vi "spot_gen_ver2.vi"(0 "amp":u32, 5 "input valid":bool, 7 "data index":u16, 9 "peak":bool, 11 "reciver_params":T1) -> (4 "PDW":u64, 6 "output valid":bool, 15 "erprr out":bool)   [LabVIEW 2021]
uses:
  FPGA/reciver params.ctl
  <vilib>/rvi/Memory/Memory_Emulation/nirvimemoryFastEmulation.vi
  <vilib>/rvi/Memory/Memory_Emulation/nirvimemoryEmulation.vi
  <vilib>/rvi/Emulation/niFpgaEmulationIsFPGAContextNoSignature.vi
  <vilib>/rvi/DataTransferAndStorage/Container/Common/niFpgaContainerGetUniqueNameForEmu.vi
  <vilib>/rvi/Emulation/niFpgaProcessEmulError.vi
  <vilib>/rvi/Emulation/niFpgaSctlEmulationGetInTimedLoop.vi
  <vilib>/rvi/errors/nirviReportUnexpectedCaseInternalError (U32).vi
  <vilib>/rvi/FXPMathLib/basic elements/FxpAddSub/XNode/nifxpmath_AddSub.xnode
  <vilib>/rvi/DataTransferAndStorage/Container/XNode/niFpgaContainer.xnode
  <vilib>/rvi/FXPMathLib/sim/FxpSim.dll
  <vilib>/rvi/FXPMathLib/FxpAdd/XNode/nifxpmath_Add.xnode
  <vilib>/rvi/FXPMathLib/FxpSub/XNode/nifxpmath_Sub.xnode
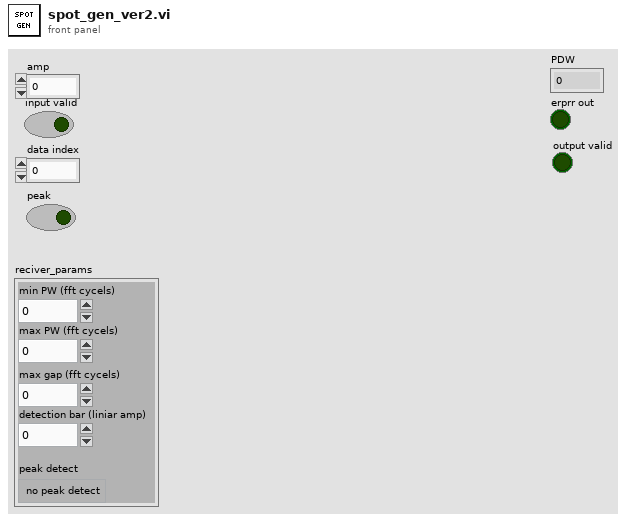
[diagram p1: front panel]
types:
  T1 = typedef "reciver params.ctl" = cluster{"min PW (fft cycels)":u16, "max PW (fft cycels)":u16, "max gap (fft cycels)":u8, "detection bar (liniar amp)":fxp<+,64,63>, "peak detect":bool}
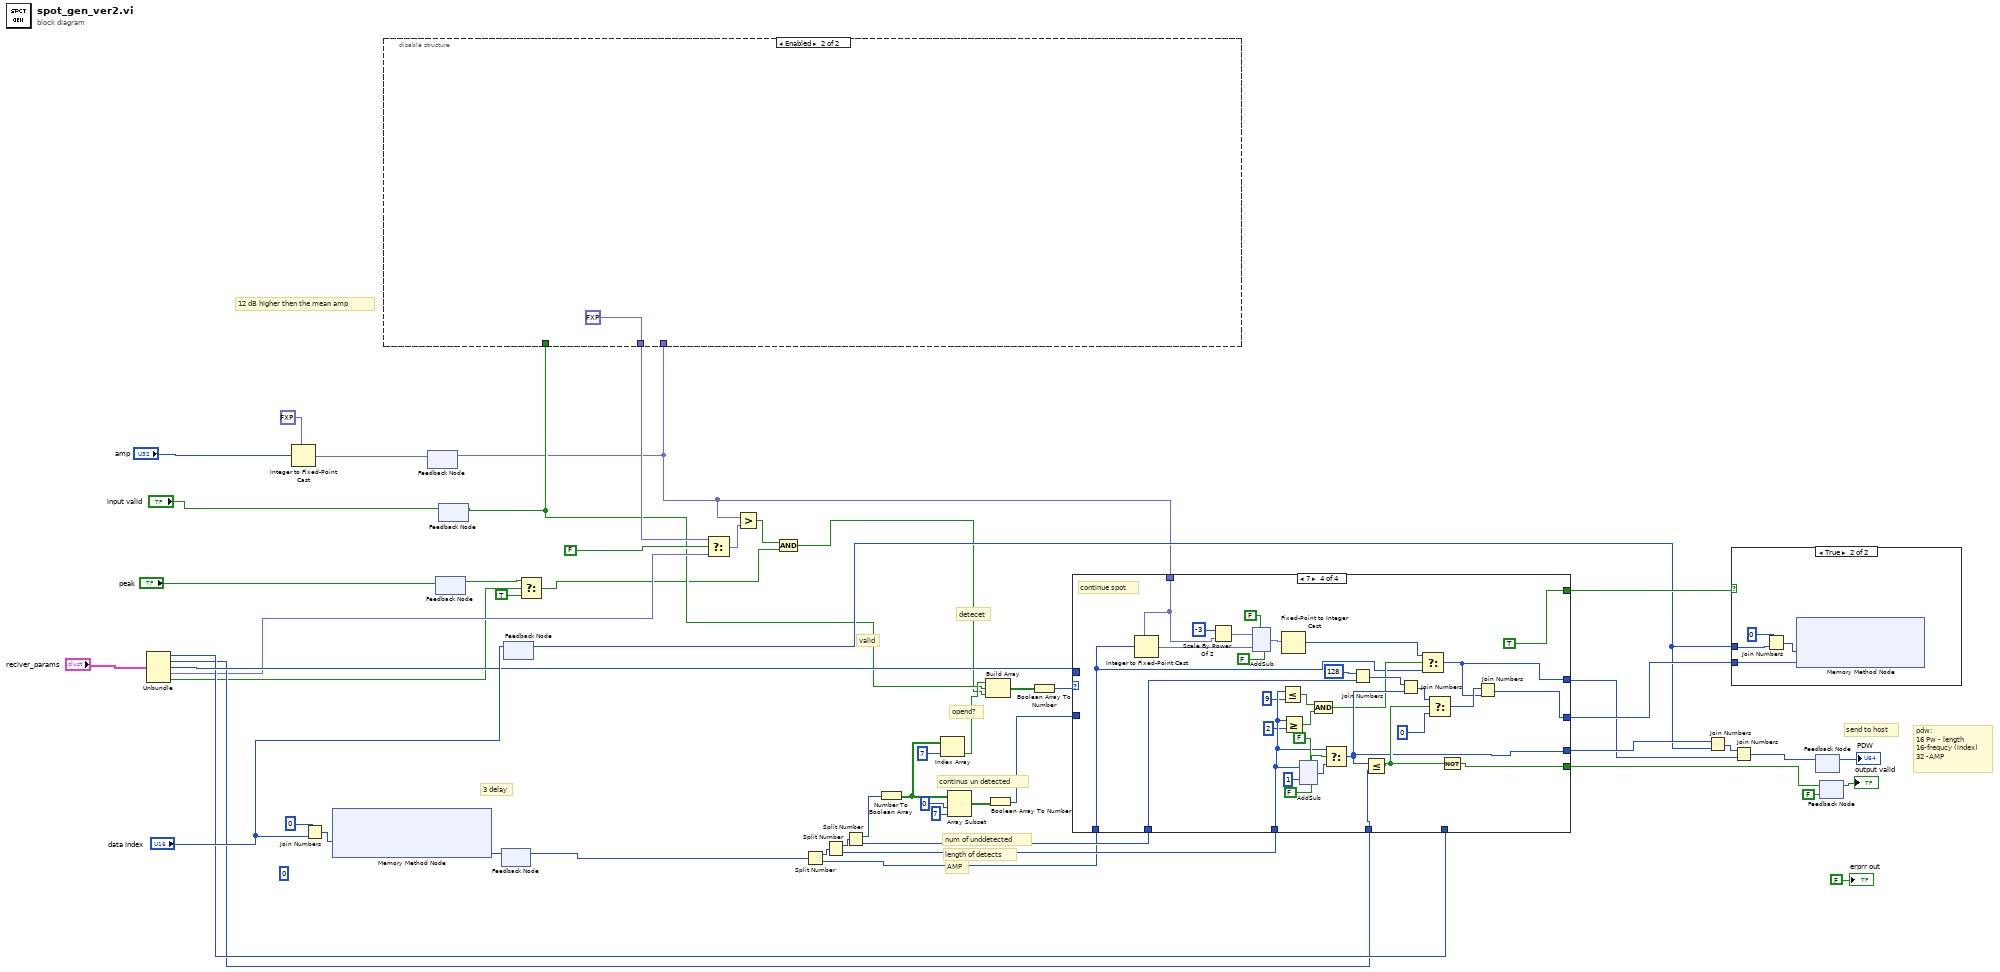
[diagram p0: block diagram]
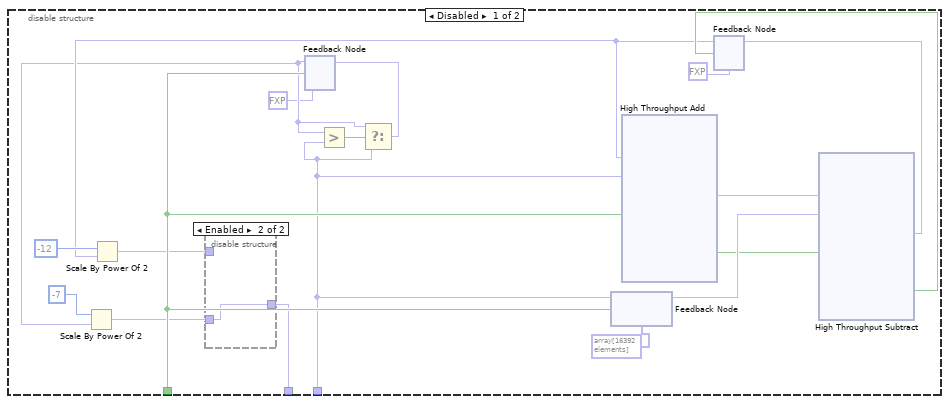
[diagram p2: hidden frame]
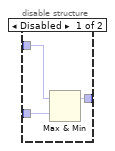
[diagram p3: hidden frame]
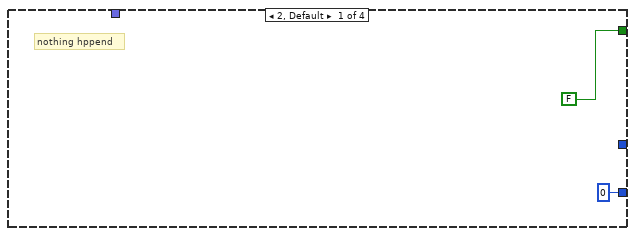
[diagram p5: hidden frame]
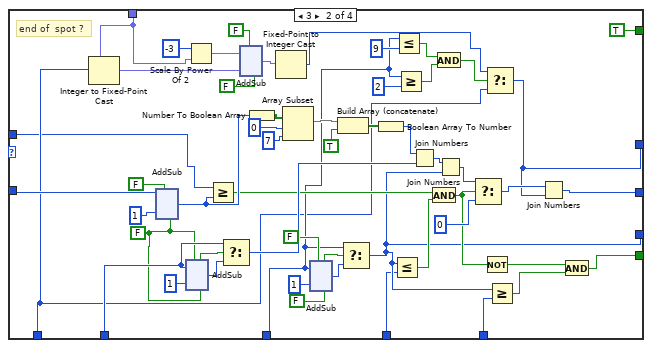
[diagram p6: hidden frame]
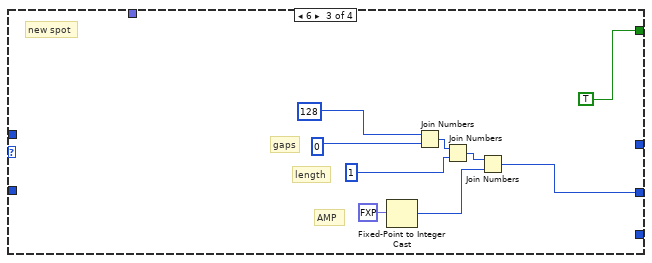
[diagram p7: hidden frame]
diagram:
  (unwired) u16 0 ("data index 2")
  # "12 dB higher then the mean amp"
  # "3 delay"
  # "AMP"
  # "pdw:\n16 Pw - length\n16-frequcy (index)\n32 -AMP"
  # "send to host"
  # "continus un detected"
  # "num of unddetected"
  # "length of detects"
  # "opend?"
  # "valid"
  # "detecet"
  n1 = Unbundle("reciver_params") -> ("min PW (fft cycels)"=w19:u16, "max PW (fft cycels)"=w18:u16, "max gap (fft cycels)"=w20:u8, "detection bar (liniar amp)"=w17:fxp<+,64,63>, "peak detect"=w1:bool)
  n2 = Integer to Fixed-Point Cast(fixed-point type=fxp<+,32,31> 0.0 ("magnitude"), integer="amp") -> (fixed-point=w6:fxp<+,32,31>)
  n3 = Join Numbers(hi=u16 0, lo="data index") -> ((hi.lo)=w24:u32)
  n4 = xnode ("Memory Method Node")("Address"=w24) -> ("Data"=w28:u64)  [unwired: 1 in, 1 out]
  n5 = feedback #1() -> (w10:fxp<+,32,31>)  [unwired: 1 in]
  n6 = feedback-in #1(w6) -> ()
  n7 = feedback #2() -> (w3:bool)  [unwired: 1 in]
  n8 = feedback-in #2("peak") -> ()
  n9 = feedback #3() -> (w11:bool)  [unwired: 1 in]
  n10 = disable-structure shown="Enabled" {
    disable-tunnel: w11 -> [w64 _]
    disable-tunnel: [w58 fxp<+,32,31> 0.0 ("magnitude")] -> w14
    disable-tunnel: w10 -> [w54 _]
    frame Disabled {
      n11 = feedback #4(fxp<+,32,31> 0.0 ("magnitude")) -> (w59:fxp<+,32,31>)
      n12 = Scale By Power Of 2(n=i8 -7 ("x"), x=w59) -> (x*2^n=w57:fxp<+,32,31>)
      n13 = Greater?(x=w59, y=w54) -> (0:w63:bool)
      n14 = Select(t=w59, s=w63, f=w54) -> (s? t:f=w61:fxp<+,32,31>)
      n15 = feedback-in #4(w61, w64) -> ()
      n16 = feedback #5(fxp<+,32,31>[] array[16392 elements]) -> (w70:fxp<+,32,31>)
      n17 = feedback-in #5(w54, w64) -> ()
      n18 = feedback #6(fxp<+,32,31> 0.0 ("s")) -> (w62:fxp<+,47,46>)
      n19 = Scale By Power Of 2(n=i8 -12 ("x"), x=w62) -> (x*2^n=w56:fxp<+,47,46>)
      n20 = disable-structure shown="Enabled" {
        disable-tunnel: [w75 w76] -> w58
        disable-tunnel: w57 -> [w74 w76]
        disable-tunnel: w56 -> [w73 _]
        frame Disabled {
          n21 = Max & Min(x=w73, y=w74) -> (max(x,y)=w75:fxp<+,47,46>)  [unwired: 1 out]
        }
        frame Enabled {
        }
      }
      n22 = xnode "High Throughput Add"("x"=w62, "y"=w54, "input valid"=w64) -> ("x+y"=w69:fxp<+,47,46>, "output valid"=w65:bool)  [unwired: 1 in, 1 out]
      n23 = xnode "High Throughput Subtract"("x"=w69, "y"=w70, "input valid"=w65) -> ("x-y"=w68:fxp<+,47,46>, "output valid"=w66:bool)  [unwired: 1 in, 1 out]
      n24 = feedback-in #6(w68, w66) -> ()
    }
    frame Enabled {
    }
  }
  n25 = feedback-in #3("input valid") -> ()
  n26 = feedback #7() -> (w27:u64)  [unwired: 1 in]
  n27 = feedback-in #7(w28) -> ()
  n28 = feedback #8() -> (w30:u16)  [unwired: 1 in]
  n29 = feedback-in #8("data index") -> ()
  n30 = Select(t=w3, s=w1, f=TRUE) -> (s? t:f=w4:bool)
  n31 = Select(t=w14, s=FALSE, f=w17) -> (s? t:f=w15:fxp<+,64,63>)
  n32 = Greater?(x=w10, y=w15) -> (0:w9:bool)
  n33 = And(x=w9, y=w4) -> (x .and. y?=w8:bool)
  n34 = Split Number(x=w27) -> (hi(x)=w34:u32, lo(x)=w33:u32)
  n35 = Split Number(x=w34) -> (hi(x)=w53:u16, lo(x)=w44:u16)
  n36 = Split Number(x=w53) -> (hi(x)=w52:u8, lo(x)=w41:u8)
  n37 = Number To Boolean Array(number=w52) -> (Boolean array=w46:bool[])
  n38 = Index Array(array=w46, index=7) -> (element=w35:bool)
  n39 = Array Subset(array=w46, index=0, length=7) -> (w49:bool[])
  n40 = Build Array(w35, w11, w8) -> (w48:bool[])
  n41 = Boolean Array To Number(Boolean array=w49) -> (number=w43:u8)
  n42 = Boolean Array To Number(Boolean array=w48) -> (number=w47:u8)
  n43 = case shown="7" w47 {
    tunnel: w44 -> [_ w87 _ w363]
    tunnel: w43 -> [_ w129 _ _]
    tunnel: [u64 0 ("Data") w99 w349 w367] -> w42
    tunnel: [FALSE TRUE TRUE TRUE] -> w40
    tunnel: w41 -> [_ w119 _ w382]
    tunnel: [_ w102 _ w376] -> w38
    tunnel: [_ w101 _ w375] -> w39
    tunnel: w33 -> [_ w84 _ w358]
    tunnel: w10 -> [_ w92 _ w370]
    tunnel: [_ w83 _ w356] -> w32
    tunnel: w20 -> [_ w82 _ _]
    tunnel: w19 -> [_ w81 _ _]
    tunnel: w18 -> [_ w80 _ w357]
    frame 2, Default {
      # "nothing hppend"
    }
    frame 3 {
      w108 = FALSE ("carry-in")
      # "end of  spot ?"
      n44 = Integer to Fixed-Point Cast(fixed-point type=w92, integer=w84) -> (fixed-point=w94:fxp<+,32,31>)
      n45 = xnode "AddSub"("x"=w129, "y"=u8 1, "carry-in"=w108, "use zero instead of x"=FALSE) -> ("s"=w130:u8)  [unwired: 1 out]
      n46 = Scale By Power Of 2(n=i16 -3, x=w92) -> (x*2^n=w95:fxp<+,32,31>)
      n47 = xnode "AddSub"("x"=w119, "y"=u8 1, "carry-in"=w108, "use zero instead of x"=w108) -> ("s"=w120:u8, "carry-out"=w121:bool)
      n48 = Greater Or Equal?(x=w82, y=w130) -> (x >= y?=w110:bool)
      n49 = Select(t=w119, s=w121, f=w120) -> (s? t:f=w118:u8)
      n50 = xnode "AddSub"("x"=w95, "y"=w94, "carry-in"=FALSE, "use zero instead of x"=FALSE) -> ("s"=w93:fxp<+,32,31>)  [unwired: 1 out]
      n51 = Number To Boolean Array(number=w130) -> (Boolean array=w126:bool[])
      n52 = Fixed-Point to Integer Cast(1:w93) -> (0:w85:u32)
      n53 = Array Subset(array=w126, index=0, length=7) -> (w105:bool[])
      n54 = xnode "AddSub"("x"=w87, "y"=u16 1, "carry-in"=FALSE, "use zero instead of x"=FALSE) -> ("s"=w115:u16, "carry-out"=w116:bool)
      n55 = Build Array (concatenate)(w105, TRUE) -> (w125:bool[])
      n56 = Select(t=w87, s=w116, f=w115) -> (s? t:f=w101:u16)
      n57 = Boolean Array To Number(Boolean array=w125) -> (number=w124:u8)
      n58 = Less Or Equal?(x=w101, y=w80) -> (x <= y?=w107:bool)
      n59 = Less Or Equal?(x=w87, y=u16 9) -> (x <= y?=w90:bool)
      n60 = Greater Or Equal?(x=w87, y=u16 2) -> (x >= y?=w91:bool)
      n61 = Join Numbers(hi=w124, lo=w118) -> ((hi.lo)=w131:u16)
      n62 = And(x=w110, y=w107) -> (x .and. y?=w109:bool)
      n63 = And(x=w90, y=w91) -> (x .and. y?=w86:bool)
      n64 = Join Numbers(hi=w131, lo=w101) -> ((hi.lo)=w114:u32)
      n65 = Select(t=w114, s=w109, f=u32 0 ("Data")) -> (s? t:f=w100:u32)
      n66 = Not(x=w109) -> (.not. x?=w104:bool)
      n67 = Select(t=w85, s=w86, f=w84) -> (s? t:f=w83:u32)
      n68 = Greater Or Equal?(x=w101, y=w81) -> (x >= y?=w103:bool)
      n69 = Join Numbers(hi=w100, lo=w83) -> ((hi.lo)=w99:u64)
      n70 = And(x=w104, y=w103) -> (x .and. y?=w102:bool)
    }
    frame 6 {
      # "gaps"
      # "length"
      # "AMP"
      # "new spot"
      n71 = Fixed-Point to Integer Cast(1:fxp<+,32,31> 0.0 ("fixed-point")) -> (0:w348:u32)
      n72 = Join Numbers(hi=u8 128, lo=u8 0 ("hi")) -> ((hi.lo)=w355:u16)
      n73 = Join Numbers(hi=w355, lo=u16 1 ("hi")) -> ((hi.lo)=w350:u32)
      n74 = Join Numbers(hi=w350, lo=w348) -> ((hi.lo)=w349:u64)
    }
    frame 7 {
      # "continue spot"
      n75 = Integer to Fixed-Point Cast(fixed-point type=w370, integer=w358) -> (fixed-point=w369:fxp<+,32,31>)
      n76 = Scale By Power Of 2(n=i16 -3, x=w370) -> (x*2^n=w371:fxp<+,32,31>)
      n77 = xnode "AddSub"("x"=w371, "y"=w369, "carry-in"=FALSE, "use zero instead of x"=FALSE) -> ("s"=w366:fxp<+,32,31>)  [unwired: 1 out]
      n78 = Less Or Equal?(x=w363, y=u16 9) -> (x <= y?=w364:bool)
      n79 = Fixed-Point to Integer Cast(1:w366) -> (0:w359:u32)
      n80 = Greater Or Equal?(x=w363, y=u16 2) -> (x >= y?=w365:bool)
      n81 = xnode "AddSub"("x"=w363, "y"=u16 1, "carry-in"=FALSE, "use zero instead of x"=FALSE) -> ("s"=w383:u16, "carry-out"=w384:bool)
      n82 = And(x=w364, y=w365) -> (x .and. y?=w360:bool)
      n83 = Select(t=w363, s=w384, f=w383) -> (s? t:f=w375:u16)
      n84 = Join Numbers(hi=u8 128, lo=w382) -> ((hi.lo)=w386:u16)
      n85 = Less Or Equal?(x=w375, y=w357) -> (x <= y?=w377:bool)
      n86 = Join Numbers(hi=w386, lo=w375) -> ((hi.lo)=w381:u32)
      n87 = Select(t=w359, s=w360, f=w358) -> (s? t:f=w356:u32)
      n88 = Select(t=w381, s=w377, f=u32 0 ("Data")) -> (s? t:f=w368:u32)
      n89 = Not(x=w377) -> (.not. x?=w376:bool)
      n90 = Join Numbers(hi=w368, lo=w356) -> ((hi.lo)=w367:u64)
    }
  }
  n91 = Join Numbers(hi=w39, lo=w30) -> ((hi.lo)=w37:u32)
  n92 = case shown="True" w40 {
    tunnel: w30 -> [_ w505]
    tunnel: w42 -> [_ w507]
    frame False {
    }
    frame True {
      n93 = Join Numbers(hi=u16 0, lo=w505) -> ((hi.lo)=w504:u32)
      n94 = xnode ("Memory Method Node")("Address"=w504, "Data"=w507) -> ()  [unwired: 1 in, 1 out]
    }
  }
  n95 = Join Numbers(hi=w37, lo=w32) -> ((hi.lo)=w23:u64)
  n96 = feedback #9() -> (→"PDW":u64)  [unwired: 1 in]
  n97 = feedback-in #9(w23) -> ()
  n98 = feedback #10(FALSE) -> (→"output valid":bool)
  n99 = feedback-in #10(w38) -> ()
  "erprr out" <- FALSE ("erprr out")
